vi "Teleop.vi"(10 "Match Info":T1={"Autonomous Elapsed Seconds"=0.0, "TeleOp Elapsed Seconds"=0.0, "Disabled Elapsed Seconds"=0.0, "Visited Autonomous"=FALSE, "Visited TeleOp"=FALSE, "Visited Disabled"=FALSE, "Autonomous Settings"={"Autonomous Style"=enum."Independent", "VI Refnum"=refnum}}, 11 "Call Context":T2) -> ()   [LabVIEW 2017]
doc: "This VI is called for each TeleOp packet received from the DS where the robot is not disabled. It is often used to read from the joysticks and update I/O or to update setpoints for timed control loops. It should complete and return within 20 milliseconds or it may miss DS packets."
uses:
  <vilib>/Rock Robotics/WPI/DriverStation/WPI_DriverStationDerivedRobotMode.ctl
  <vilib>/Rock Robotics/WPI/DriverStation/WPI_DriverStationMatch Info.ctl
  <vilib>/Rock Robotics/WPI/Utilities/WPI_GetSetVariantRefNum.vi
  <vilib>/Rock Robotics/Network Tables/NT Write Boolean Array.vi
  <vilib>/Rock Robotics/Network Tables/NT Write Numeric Array.vi
  <vilib>/Rock Robotics/Network Tables/NT Read Boolean.vi
  <vilib>/Rock Robotics/Network Tables/NT Read Number.vi
panel:
  out "Sample Slider 0":dbl(slide) scale=0.0..5.0
  out "Sample Boolean 1":bool
  out "Sample Boolean 0":bool
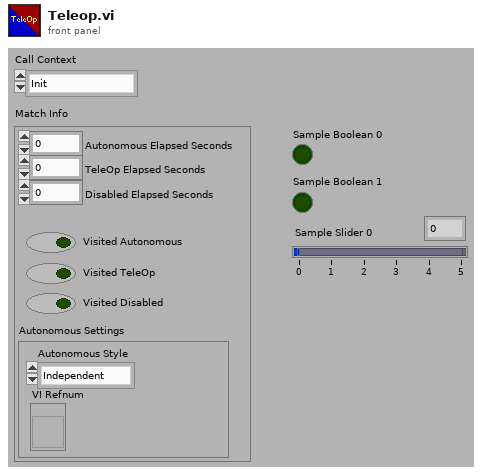
[diagram p1: front panel]
types:
  T1 = typedef "WPI_DriverStationMatch Info.ctl" = cluster{"Autonomous Elapsed Seconds":dbl, "TeleOp Elapsed Seconds":dbl, "Disabled Elapsed Seconds":dbl, "Visited Autonomous":bool, "Visited TeleOp":bool, "Visited Disabled":bool, "Autonomous Settings":cluster{"Autonomous Style":enum16{"Iterative", "Independent"}, "VI Refnum":refnum<vi>}}
  T2 = typedef "WPI_DriverStationDerivedRobotMode.ctl" = enum16{"Init", "Execute", "Stop"}
  T3 = typedef "WPI_RobotDriveDevRef.ctl" = cluster{"DevStatus":errorcluster, "Motors[]":T4[], "Square Inputs":bool, "Max Output":dbl}
  T4 = typedef "WPI_MotorControlDeviceRef.ctl" = cluster{"DeviceStatus":errorcluster, "Type":T5, "PWM":cluster{"PWM Channel":T6, "DeadBand":T7}, "CAN":cluster{"Device Number":u8, "SetOutput VI Ref":variant, "GetOutput VI Ref":variant, "Enable VI Ref":variant, "Disable VI Ref":variant, "Data":variant}, "Invert":bool, "DIO PWM":cluster{"PWM \"Enable\" Channel":T6, "DIOChannel":T8, "PWM Rate":dbl}}
  T5 = typedef "WPI_MotorControlType.ctl" = enum16{"PWM", "CAN", "DIO PWM"}
  T6 = typedef "FPGA_DIOPWMChannel.ctl" = enum8{"PWM 0", "PWM 1", "PWM 2", "PWM 3", "PWM 4", "PWM 5", "PWM 6", "PWM 7", "PWM 8", "PWM 9", "PWM MXP 0", "PWM MXP 1", "PWM MXP 2", "PWM MXP 3", "PWM MXP 4", "PWM MXP 5", "PWM MXP 6", "PWM MXP 7", "PWM MXP 8", "PWM MXP 9", "Invalid"}
  T7 = typedef "WPI_PWMDeadband.ctl" = cluster{"Name":string, "maxPositivePwm":i32, "minPositivePwm":i32, "centerPwm":i32, "maxNegativePwm":i32, "minNegativePwm":i32, "angularRange":u16}
  T8 = typedef "FPGA_DIOChannel.ctl" = enum8{"DIO 0", "DIO 1", "DIO 2", "DIO 3", "DIO 4", "DIO 5", "DIO 6", "DIO 7", "DIO 8", "DIO 9", "DIO MXP 0", "DIO MXP 1", "DIO MXP 2", "DIO MXP 3", "DIO MXP 4", "DIO MXP 5", "DIO MXP 6", "DIO MXP 7", "DIO MXP 8", "DIO MXP 9", "DIO MXP 10", "DIO MXP 11", "DIO MXP 12", "DIO MXP 13", "DIO MXP 14", "DIO MXP 15", "SPI Port CS1", "SPI Port CS2", "SPI Port CS3", "SPI Port MISO", "SPI Port MOSI", "Invalid"}
  T9 = typedef "WPI_JoystickDevRef.ctl" = cluster{"Device":T10}
  T10 = typedef "WPI_JoystickDeviceEnum.ctl" = enum16{"USB 0", "USB 1", "USB 2", "USB 3", "USB 4", "USB 5"}
  T11 = typedef "WPI_SwitchDevRef.ctl" = cluster{"DevStatus":errorcluster, "DIO Channel":T8, "CntIndex":T12, "Normally Closed":bool}
  T12 = typedef "FPGA_CounterCtrSystemIndex.ctl" = enum8{"Ctr 0", "Ctr 1", "Ctr 2", "Ctr 3", "Ctr 4", "Ctr 5", "Ctr 6", "Ctr 7", "Invalid"}
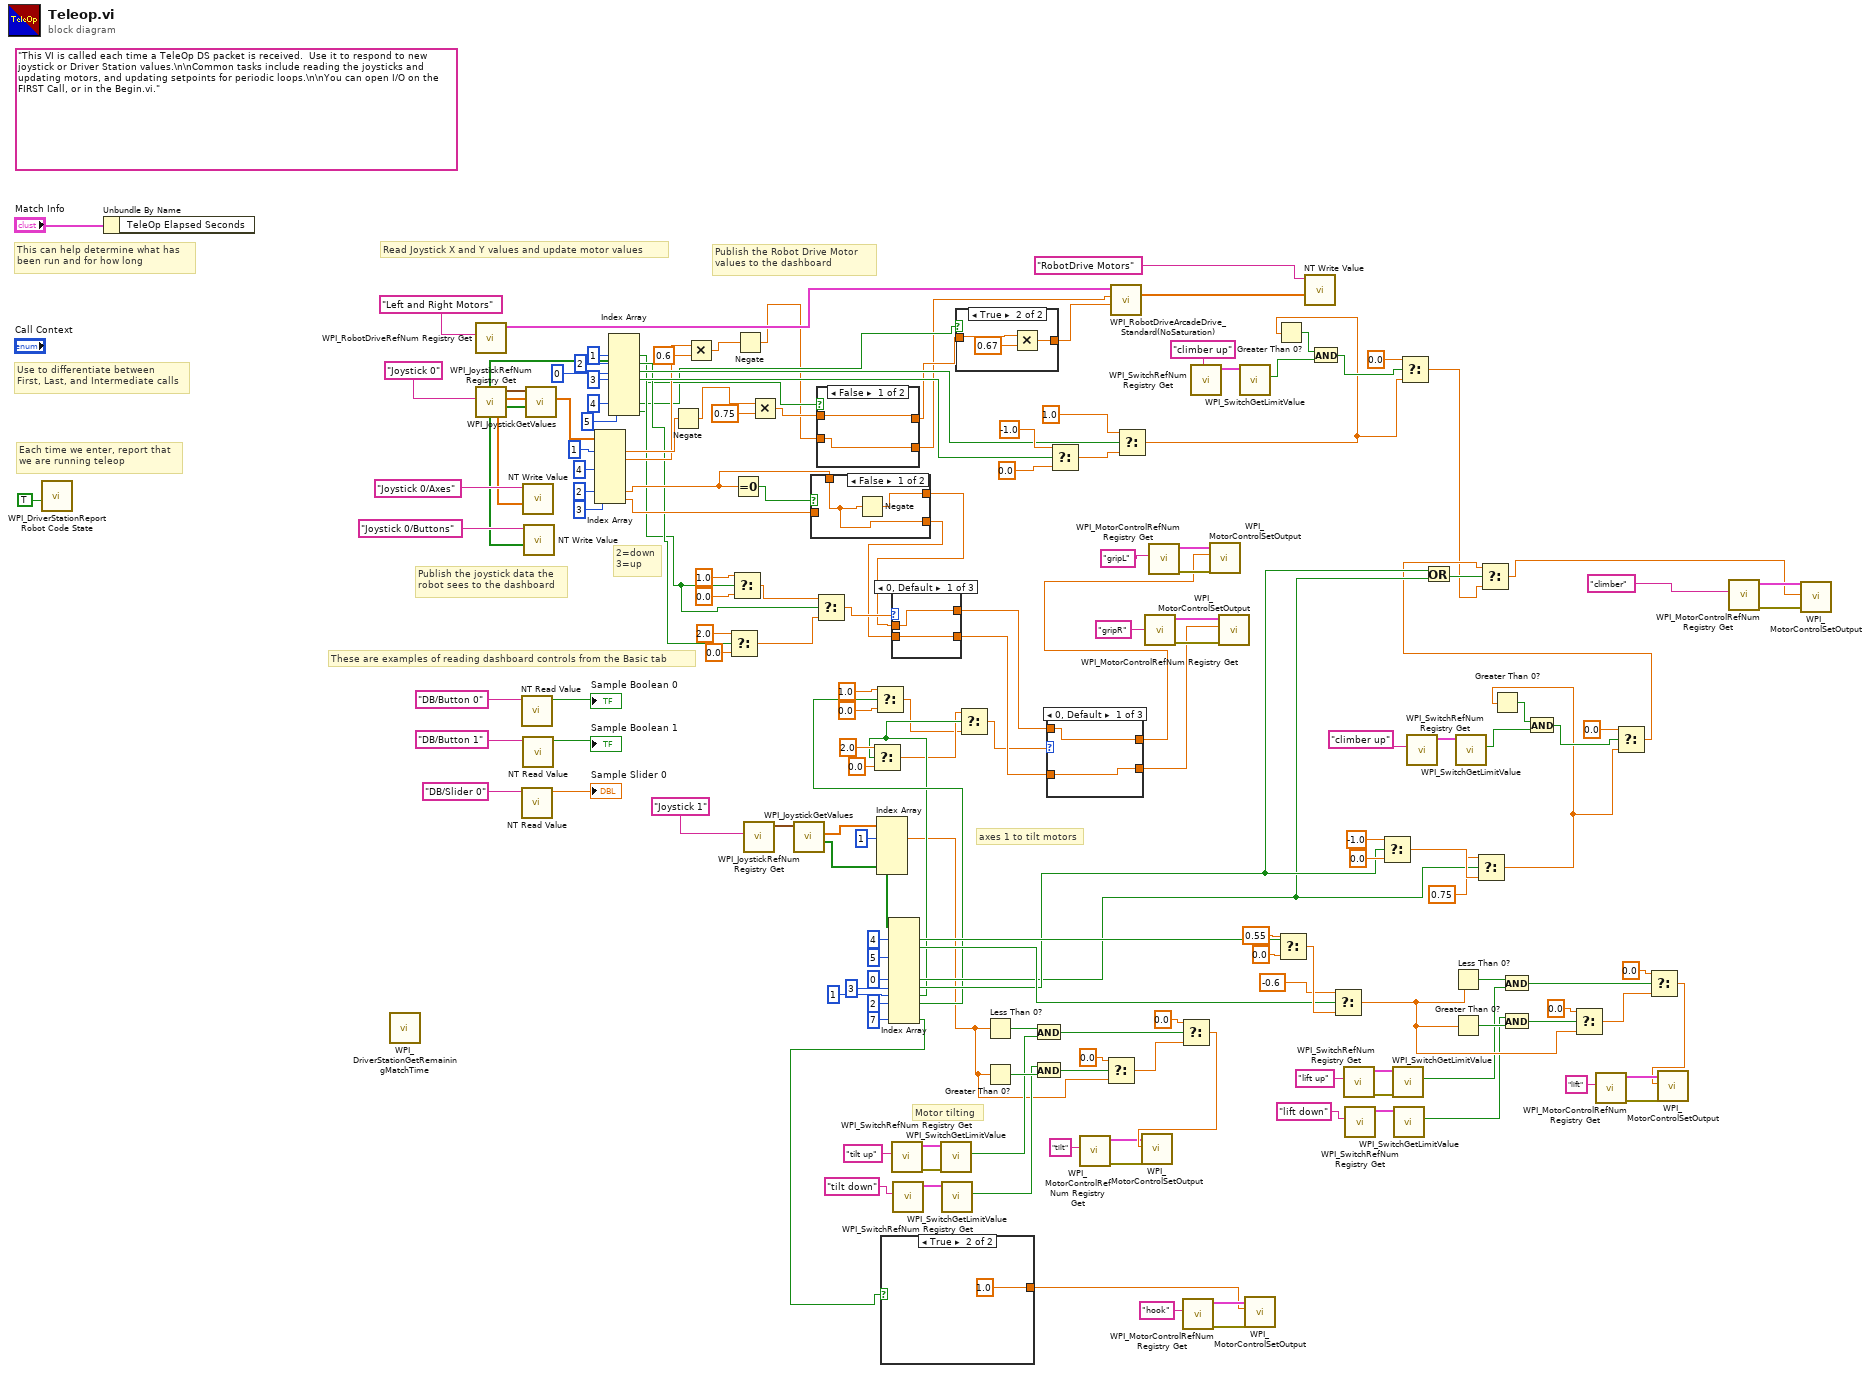
[diagram p0: block diagram]
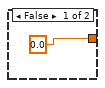
[diagram p2: hidden frame]
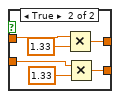
[diagram p4: hidden frame]
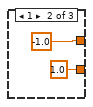
[diagram p5: hidden frame]
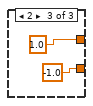
[diagram p6: hidden frame]
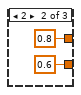
[diagram p7: hidden frame]
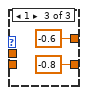
[diagram p8: hidden frame]
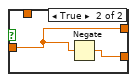
[diagram p9: hidden frame]
diagram:
  (unwired) "This VI is called each time a TeleOp DS packet is received.  Use it to respond to new joystick or Driver Station values.\n\nCommon tasks include reading the joysticks and updating motors, and updating setpoints for periodic loops.\n\nYou can open I/O on the FIRST Call, or in the Begin.vi."
  # "Motor tilting"
  # "axes 1 to tilt motors"
  # "2=down\n3=up"
  # "These are examples of reading dashboard controls from the Basic tab"
  # "Publish the Robot Drive Motor\nvalues to the dashboard"
  # "Publish the joystick data the\nrobot sees to the dashboard"
  # "Each time we enter, report that\nwe are running teleop"
  # "Use to differentiate between\nFirst, Last, and Intermediate calls"
  # "This can help determine what has\nbeen run and for how long"
  # "Read Joystick X and Y values and update motor values"
  n1 = call <vilib>:"WPI_DriverStationReport Robot Code State.vi"("TeleOp"=TRUE ("Autonomous")) -> ()  [unwired: 10 in, 1 out]
  n2 = Unbundle By Name("Match Info") -> ()  [unwired: 1 out]
  n3 = call <vilib>:"WPI_DriverStationGetRemainingMatchTime.vi"() -> ()  [unwired: 10 in, 2 out]
  n4 = call <vilib>:"WPI_RobotDriveRefNum Registry Get.vi"("refnum name"="Left and Right Motors") -> ("RobotDriveDevRef"=w166:T3)  [unwired: 1 in, 9 out]
  n5 = call <vilib>:"WPI_JoystickRefNum Registry Get.vi"("refnum name"="Joystick 0") -> ("JoystickDevRef"=w164:T9)  [unwired: 1 in, 9 out]
  n6 = call-poly <vilib>:"NT Read Value.vi"("Name"="DB/Button 0" ("refnum name")) -> ("Boolean"=→"Sample Boolean 0":bool)  [unwired: 9 in, 1 out]
  n7 = call-poly <vilib>:"NT Read Value.vi"("Name"="DB/Slider 0" ("refnum name")) -> ("Numeric"=→"Sample Slider 0":dbl)  [unwired: 9 in, 1 out]
  n8 = call-poly <vilib>:"NT Read Value.vi"("Name"="DB/Button 1" ("refnum name")) -> ("Boolean"=→"Sample Boolean 1":bool)  [unwired: 9 in, 1 out]
  n9 = call <vilib>:"WPI_JoystickGetValues.vi"("JoystickDevRef"=w164) -> ("Buttons"=w147:bool[], "Axes"=w160:dbl[])  [unwired: 6 in, 3 out]
  n10 = call-poly <vilib>:"NT Write Value.vi"("Numeric Array"=w160, "Name"="Joystick 0/Axes") -> ()  [unwired: 9 in, 1 out]
  n11 = call-poly <vilib>:"NT Write Value.vi"("Boolean Array"=w147, "Name"="Joystick 0/Buttons") -> ()  [unwired: 9 in, 1 out]
  n12 = Index Array(array=w160, index #1=1 ("index"), index #2=4 ("index"), index #6=2 ("index"), index #7=3 ("index")) -> (element #1=w134:dbl, element #2=w125:dbl, element #6=w128:dbl, element #7=w129:dbl)  [unwired: 3 in, 3 out]
  n13 = Index Array(array=w147, index #1=1 ("index"), index #2=2 ("index"), index #3=0 ("index"), index #4=3 ("index"), index #7=4 ("index"), index #8=5 ("index")) -> (element #1=w54:bool, element #2=w57:bool, element #3=w135:bool, element #4=w142:bool, element #7=w39:bool, element #8=w43:bool)  [unwired: 2 in, 2 out]
  n14 = Negate(x=w134) -> (-x=w127:dbl)
  n15 = Multiply(x=w125, y=0.6) -> (x*y=w123:dbl)
  n16 = Select(t=2.0, s=w57, f=0.0) -> (s? t:f=w58:dbl)
  n17 = Select(t=1.0, s=w54, f=0.0) -> (s? t:f=w59:dbl)
  n18 = Equal To 0?(x=w128) -> (x = 0?=w130:bool)
  n19 = Negate(x=w123) -> (-x=w38:dbl)
  n20 = call <vilib>:"WPI_JoystickRefNum Registry Get.vi"("refnum name"="Joystick 1") -> ("JoystickDevRef"=w150:T9)  [unwired: 1 in, 9 out]
  n21 = Multiply(x=w127, y=0.75) -> (x*y=w42:dbl)
  n22 = call <vilib>:"WPI_JoystickGetValues.vi"("JoystickDevRef"=w150) -> ("Buttons"=w93:bool[], "Axes"=w149:dbl[])  [unwired: 6 in, 3 out]
  n23 = case shown="False" w130 {
    tunnel: [w170 w172] -> w52
    tunnel: w129 -> [_ w172]
    tunnel: w128 -> [w169 _]
    tunnel: [w169 w171] -> w51
    frame False {
      n24 = Negate(x=w169) -> (-x=w170:dbl)
    }
    frame True {
      n25 = Negate(x=w172) -> (-x=w171:dbl)
    }
  }
  n26 = Select(t=w59, s=w54, f=w58) -> (s? t:f=w53:dbl)
  n27 = case shown="False" w43 {
    tunnel: w42 -> [w174 w180]
    tunnel: [w174 w178] -> w41
    tunnel: w38 -> [w173 w176]
    tunnel: [w173 w175] -> w37
    frame False {
    }
    frame True {
      n28 = Multiply(x=w180, y=1.33) -> (x*y=w178:dbl)
      n29 = Multiply(x=w176, y=1.33) -> (x*y=w175:dbl)
    }
  }
  n30 = Index Array(array=w149, index #1=1 ("index")) -> (element #1=w10:dbl)  [unwired: 4 in, 4 out]
  n31 = Index Array(array=w93, index #1=4 ("index"), index #2=5 ("index"), index #6=0 ("index"), index #7=3 ("index"), index #8=1 ("index"), index #9=2 ("index"), index #11=7 ("index")) -> (element #1=w90:bool, element #2=w89:bool, element #6=w70:bool, element #7=w71:bool, element #8=w30:bool, element #9=w31:bool, element #11=w2:bool)  [unwired: 4 in, 4 out]
  n32 = Select(t=2.0, s=w30, f=0.0) -> (s? t:f=w8:dbl)
  n33 = Select(t=1.0, s=w31, f=0.0) -> (s? t:f=w7:dbl)
  n34 = case shown="True" w2 {
    tunnel: [0.0 ("Output") 1.0 ("Output")] -> w1
    frame False {
    }
    frame True {
    }
  }
  n35 = case shown="0, Default" w53 {
    tunnel: [w184 0.8 ("upper limit") -0.6 ("upper limit")] -> w48
    tunnel: w52 -> [w184 _ _]
    tunnel: [w183 0.6 ("upper limit") -0.8 ("upper limit")] -> w46
    tunnel: w51 -> [w183 _ _]
    frame 0, Default {
    }
    frame 2 {
    }
    frame 1 {
    }
  }
  n36 = call <vilib>:"WPI_SwitchRefNum Registry Get.vi"("refnum name"="tilt up") -> ("error out"=w27:errorcluster, "SwitchDevRef"=w26:T11)  [unwired: 9 in]
  n37 = call <vilib>:"WPI_SwitchRefNum Registry Get.vi"("refnum name"="tilt down") -> ("SwitchDevRef"=w25:T11)  [unwired: 9 in, 1 out]
  n38 = call <vilib>:"WPI_SwitchGetLimitValue.vi"("error in (no error)"=w27, "SwitchDevRef"=w26) -> ("Switch Pressed"=w12:bool)  [unwired: 7 in, 2 out]
  n39 = call <vilib>:"WPI_SwitchGetLimitValue.vi"("SwitchDevRef"=w25) -> ("Switch Pressed"=w13:bool)  [unwired: 8 in, 2 out]
  n40 = case shown="True" w39 {
    tunnel: w41 -> [w189 w192]
    tunnel: [w189 w190] -> w40
    frame False {
    }
    frame True {
      n41 = Multiply(x=w192, y=0.67) -> (x*y=w190:dbl)
    }
  }
  n42 = Select(t=w8, s=w30, f=w7) -> (s? t:f=w29:dbl)
  n43 = Less Than 0?(x=w10) -> (x < 0?=w17:bool)
  n44 = Greater Than 0?(x=w10) -> (x > 0?=w18:bool)
  n45 = And(x=w17, y=w12) -> (x .and. y?=w19:bool)
  n46 = And(x=w13, y=w18) -> (x .and. y?=w20:bool)
  n47 = case shown="0, Default" w29 {
    tunnel: [w193 -1.0 ("upper limit") 1.0 ("upper limit")] -> w49
    tunnel: w48 -> [w193 _ _]
    tunnel: [w194 1.0 ("upper limit") -1.0 ("upper limit")] -> w47
    tunnel: w46 -> [w194 _ _]
    frame 0, Default {
    }
    frame 1 {
    }
    frame 2 {
    }
  }
  n48 = Select(t=-1.0, s=w142, f=0.0) -> (s? t:f=w139:dbl)
  n49 = call <vilib>:"WPI_MotorControlRefNum Registry Get.vi"("refnum name"="tilt") -> ("error out"=w21:errorcluster, "MotorControlDevRef"=w9:T4)  [unwired: 9 in]
  n50 = Select(t=0.0, s=w20, f=w10) -> (s? t:f=w14:dbl)
  n51 = call <vilib>:"WPI_RobotDriveArcadeDrive_Standard(NoSaturation).vi"("Y axis value"=w40, "X axis value"=w37, "RobotDriveDevRef"=w166) -> ("Motor Values"=w153:dbl[])  [unwired: 1 in, 7 out]
  n52 = Select(t=1.0, s=w135, f=w139) -> (s? t:f=w116:dbl)
  n53 = call <vilib>:"WPI_MotorControlRefNum Registry Get.vi"("refnum name"="gripR") -> ("error out"=w65:errorcluster, "MotorControlDevRef"=w45:T4)  [unwired: 9 in]
  n54 = call <vilib>:"WPI_MotorControlRefNum Registry Get.vi"("refnum name"="gripL") -> ("error out"=w131:errorcluster, "MotorControlDevRef"=w132:T4)  [unwired: 9 in]
  n55 = Select(t=0.0, s=w19, f=w14) -> (s? t:f=w11:dbl)
  n56 = call <vilib>:"WPI_MotorControlSetOutput.vi"("error in (no error)"=w21, "Output"=w11, "MotorControlDevRef"=w9) -> ()  [unwired: 6 in, 3 out]
  n57 = call <vilib>:"WPI_MotorControlRefNum Registry Get.vi"("refnum name"="hook") -> ("error out"=w5:errorcluster, "MotorControlDevRef"=w4:T4)  [unwired: 9 in]
  n58 = call <vilib>:"WPI_SwitchRefNum Registry Get.vi"("refnum name"="climber up") -> ("SwitchDevRef"=w122:T11)  [unwired: 9 in, 1 out]
  n59 = call <vilib>:"WPI_MotorControlSetOutput.vi"("error in (no error)"=w131, "Output"=w49, "MotorControlDevRef"=w132) -> ()  [unwired: 6 in, 3 out]
  n60 = call <vilib>:"WPI_MotorControlSetOutput.vi"("error in (no error)"=w65, "Output"=w47, "MotorControlDevRef"=w45) -> ()  [unwired: 6 in, 3 out]
  n61 = call <vilib>:"WPI_SwitchGetLimitValue.vi"("SwitchDevRef"=w122) -> ("Switch Pressed"=w120:bool)  [unwired: 8 in, 2 out]
  n62 = call <vilib>:"WPI_MotorControlSetOutput.vi"("error in (no error)"=w5, "Output"=w1, "MotorControlDevRef"=w4) -> ()  [unwired: 6 in, 3 out]
  n63 = Greater Than 0?(x=w116) -> (x > 0?=w119:bool)
  n64 = Select(t=0.55, s=w90, f=0.0) -> (s? t:f=w110:dbl)
  n65 = call-poly <vilib>:"NT Write Value.vi"("Numeric Array"=w153, "Name"="RobotDrive Motors") -> ()  [unwired: 9 in, 1 out]
  n66 = And(x=w119, y=w120) -> (x .and. y?=w117:bool)
  n67 = Select(t=-0.6, s=w89, f=w110) -> (s? t:f=w101:dbl)
  n68 = call <vilib>:"WPI_SwitchRefNum Registry Get.vi"("refnum name"="lift up") -> ("error out"=w99:errorcluster, "SwitchDevRef"=w98:T11)  [unwired: 9 in]
  n69 = call <vilib>:"WPI_SwitchRefNum Registry Get.vi"("refnum name"="lift down") -> ("SwitchDevRef"=w97:T11)  [unwired: 9 in, 1 out]
  n70 = Select(t=-1.0, s=w71, f=0.0) -> (s? t:f=w83:dbl)
  n71 = call <vilib>:"WPI_SwitchGetLimitValue.vi"("error in (no error)"=w99, "SwitchDevRef"=w98) -> ("Switch Pressed"=w95:bool)  [unwired: 7 in, 2 out]
  n72 = call <vilib>:"WPI_SwitchGetLimitValue.vi"("SwitchDevRef"=w97) -> ("Switch Pressed"=w94:bool)  [unwired: 8 in, 2 out]
  n73 = Select(t=0.0, s=w117, f=w116) -> (s? t:f=w67:dbl)
  n74 = call <vilib>:"WPI_SwitchRefNum Registry Get.vi"("refnum name"="climber up") -> ("SwitchDevRef"=w81:T11)  [unwired: 9 in, 1 out]
  n75 = Or(x=w71, y=w70) -> (x .or. y?=w69:bool)
  n76 = Less Than 0?(x=w101) -> (x < 0?=w105:bool)
  n77 = Greater Than 0?(x=w101) -> (x > 0?=w106:bool)
  n78 = call <vilib>:"WPI_SwitchGetLimitValue.vi"("SwitchDevRef"=w81) -> ("Switch Pressed"=w79:bool)  [unwired: 8 in, 2 out]
  n79 = Select(t=0.75, s=w70, f=w83) -> (s? t:f=w75:dbl)
  n80 = Greater Than 0?(x=w75) -> (x > 0?=w78:bool)
  n81 = And(x=w105, y=w95) -> (x .and. y?=w107:bool)
  n82 = And(x=w94, y=w106) -> (x .and. y?=w108:bool)
  n83 = And(x=w78, y=w79) -> (x .and. y?=w76:bool)
  n84 = Select(t=0.0, s=w108, f=w101) -> (s? t:f=w102:dbl)
  n85 = call <vilib>:"WPI_MotorControlRefNum Registry Get.vi"("refnum name"="lift") -> ("error out"=w113:errorcluster, "MotorControlDevRef"=w114:T4)  [unwired: 9 in]
  n86 = Select(t=0.0, s=w76, f=w75) -> (s? t:f=w68:dbl)
  n87 = Select(t=w68, s=w69, f=w67) -> (s? t:f=w66:dbl)
  n88 = Select(t=0.0, s=w107, f=w102) -> (s? t:f=w100:dbl)
  n89 = call <vilib>:"WPI_MotorControlSetOutput.vi"("error in (no error)"=w113, "Output"=w100, "MotorControlDevRef"=w114) -> ()  [unwired: 6 in, 3 out]
  n90 = call <vilib>:"WPI_MotorControlRefNum Registry Get.vi"("refnum name"="climber") -> ("error out"=w86:errorcluster, "MotorControlDevRef"=w87:T4)  [unwired: 9 in]
  n91 = call <vilib>:"WPI_MotorControlSetOutput.vi"("error in (no error)"=w86, "Output"=w66, "MotorControlDevRef"=w87) -> ()  [unwired: 6 in, 3 out]
